vi "Read Pin.vi"(6 "Pin":u16, 8 "error in (no error)":errorcluster, 9 "Port":u16, 10 "VISA resource name":refnum<visa-resource-name>, 11 "NXP in":refnum<class "NXP.lvclass">) -> (0 "error out":errorcluster, 1 "Boolean":bool, 2 "VISA resource name 2":refnum<visa-resource-name>, 3 "NXP out":refnum<class "NXP.lvclass">)   [LabVIEW 2020, in "NXP.lvclass"]
uses:
  NXP.lvclass
panel:
  out "concatenated string":string
  out "String 2":string
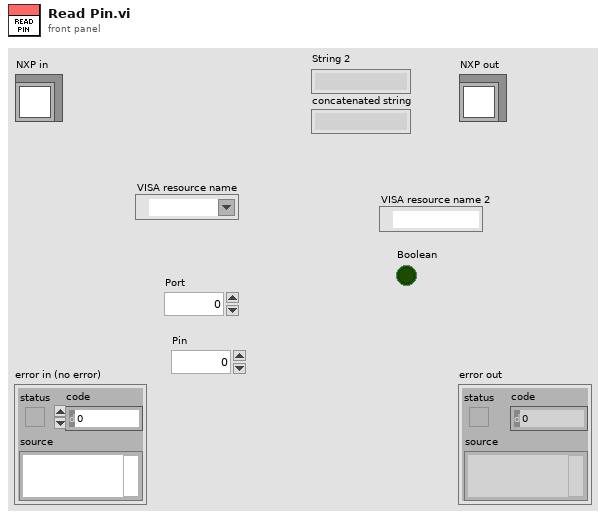
[diagram p1: front panel]
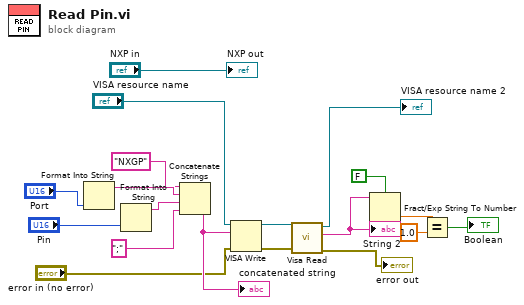
[diagram p0: block diagram]
diagram:
  n1 = Format Into String("Port") -> (resulting string=w18:string)  [unwired: 3 in, 1 out]
  n2 = Format Into String("Pin") -> (resulting string=w12:string)  [unwired: 3 in, 1 out]
  n3 = Concatenate Strings("NXGP" ("string"), w18, w12, ";" ("string")) -> (w15:string)
  "concatenated string" <- w15
  n4 = VISA Write(VISA resource name="VISA resource name", write buffer=w15, error in (no error)="error in (no error)") -> (VISA resource name out=w16:refnum<visa-resource-name>, error out=w14:errorcluster)  [unwired: 1 out]
  n5 = call "Visa Read.vi"("error in (no error)"=w14, "VISA Refnum in"=w16) -> ("error out"=→"error out":errorcluster, "String 2"=w5:string, "VISA Refnum out"=→"VISA resource name 2":refnum<visa-resource-name>)  [unwired: 7 in]
  "String 2" <- w5
  n6 = Fract/Exp String To Number(use system decimal point (T)=FALSE, string=w5) -> (number=w3:dbl)  [unwired: 2 in, 1 out]
  n7 = Equal?(x=w3, y=1.0) -> (x = y?=→"Boolean":bool)
  "NXP out" <- "NXP in"
